vi "Start.vi"(8 "error in (no error)":errorcluster, 11 "Framework in":refnum<class "Framework.lvclass">) -> (0 "error out":errorcluster, 3 "Framework out":refnum<class "Framework.lvclass">)   [LabVIEW 2017, in "DSF Core.lvlib" / "Framework.lvclass"]
uses:
  Framework.lvclass
  Framework States.ctl
  Framework.lvclass/Framework.ctl
  Interface/Dispatcher/Dispatcher Interface.lvclass
  Interface/Logging/Logging Interface.lvclass
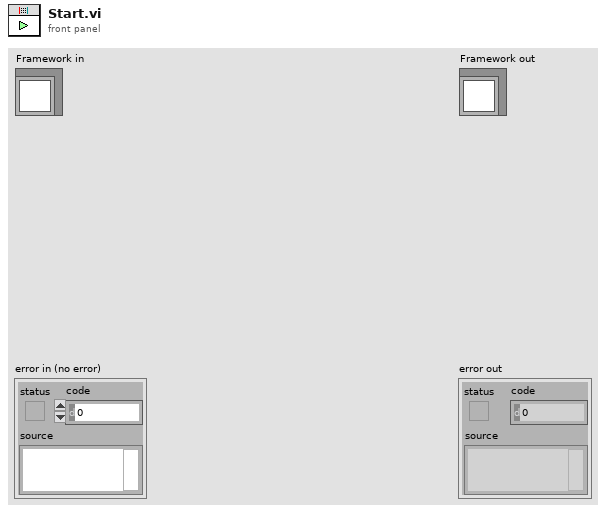
[diagram p1: front panel]
types:
  T1 = typedef "DSF Core.lvlib/Framework.lvclass/Framework States.ctl" = enum8{"Uninitialized", "Initialized", "Start", "Rx", "Tx", "Shutdown"}
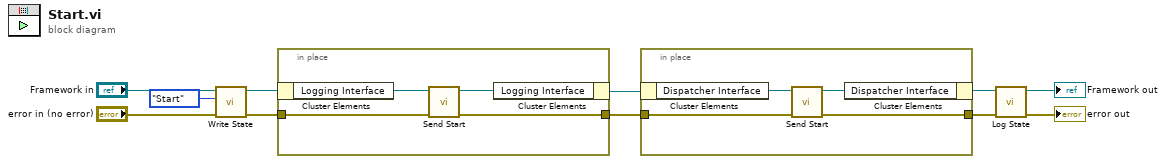
[diagram p0: block diagram]
diagram:
  n1 = call "Write State.vi"("error in (no error)"="error in (no error)", "state"=Framework_States."Start", "Framework in"="Framework in") -> ("error out"=w8:errorcluster, "Framework out"=w7:refnum<class "Framework.lvclass">)  [unwired: 7 in]
  n2 = in-place {
    in-place-border: w8 -> [w15]
    in-place-border: [w14] -> w11
    n3 = in-place-cluster #1(w7) -> ("Logging Interface"=w13:refnum<class "Logging Interface.lvclass">)
    n4 = call "Send Start.vi"("error in (no error)"=w15, "Logging Interface in"=w13) -> ("error out"=w14:errorcluster, "Logging Interface out"=w12:refnum<class "Logging Interface.lvclass">)  [unwired: 8 in]
    n5 = in-place-cluster #1("Logging Interface"=w12) -> (w10:refnum<class "Framework.lvclass">)
  }
  n6 = in-place {
    in-place-border: w11 -> [w18]
    in-place-border: [w17] -> w3
    n7 = in-place-cluster #2(w10) -> ("Dispatcher Interface"=w19:refnum<class "Dispatcher Interface.lvclass">)
    n8 = call "Send Start.vi"("error in (no error)"=w18, "Dispatcher Interface in"=w19) -> ("error out"=w17:errorcluster, "Dispatcher Interface out"=w16:refnum<class "Dispatcher Interface.lvclass">)  [unwired: 8 in]
    n9 = in-place-cluster #2("Dispatcher Interface"=w16) -> (w4:refnum<class "Framework.lvclass">)
  }
  n10 = call "Log State.vi"("error in (no error)"=w3, "Framework in"=w4) -> ("error out"=→"error out":errorcluster, "Framework out"=→"Framework out":refnum<class "Framework.lvclass">)  [unwired: 8 in]
